vi "Draw Palette.vi"(2 "Bounds  Of Picture":T1, 3 "Display Data":T3[](array[typedef])) -> (0 "Co-ordinates":T2(array[cluster]), 1 "picture":picture)   [LabVIEW 2014, in "SmartPalette.lvlib"]
uses:
  SmartPalette.lvlib
  Controls/Palette Data.ctl
  <vilib>/picture/picture.llb/imagedata.ctl
  <vilib>/Utility/miscctls.llb/LVBoundsTypeDef.ctl
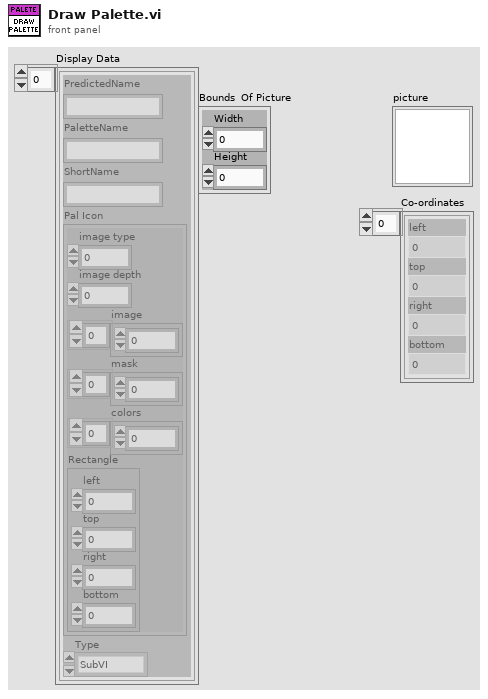
[diagram p1: front panel]
types:
  T1 = typedef "LVBoundsTypeDef.ctl" = cluster{"Width":u32, "Height":u32}
  T2 = cluster{"left":i16, "top":i16, "right":i16, "bottom":i16}[]
  T3 = typedef "SmartPalette.lvlib/Palette Data.ctl" = cluster{"PredictedName":string, "PaletteName":string, "ShortName":string, "Pal Icon":T4, "Type":enum16{"SubVI", "VI Templtate", "Function"}}
  T4 = typedef "imagedata.ctl" = cluster{"image type":i32, "image depth":i32, "image":u8[], "mask":u8[], "colors":u32[], "Rectangle":cluster{"left":i16, "top":i16, "right":i16, "bottom":i16}}
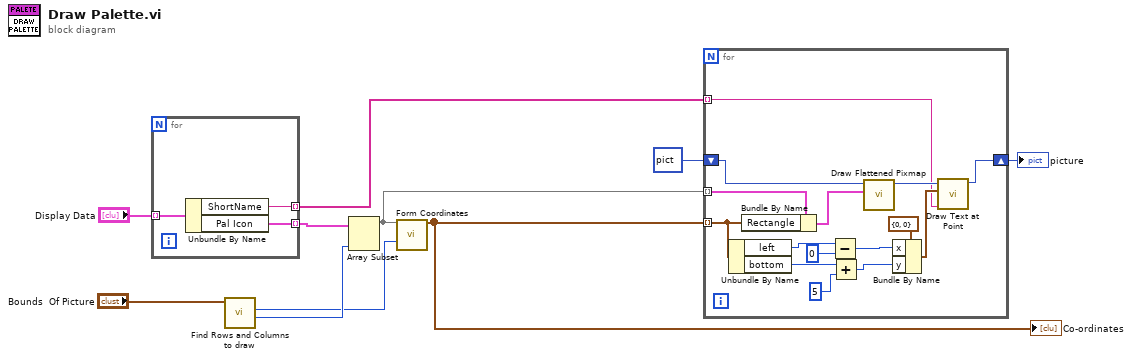
[diagram p0: block diagram]
diagram:
  n1 = for {
    tunnel: "Display Data" -> [w13] mode=indexing
    tunnel: [w12] -> w4 mode=indexing
    tunnel: [w11] -> w8 mode=indexing
    n2 = Unbundle By Name(w13) -> ("ShortName"=w11:string, "Pal Icon"=w12:T4)
  }
  n3 = call "Find Rows and Columns to draw.vi"("Bounds  Of Picture"="Bounds  Of Picture") -> ("Total"=w2:u32, "Col"=w1:u32)  [unwired: 8 in, 1 out]
  n4 = Array Subset(array=w4, length=w2) -> (w5:T4[])  [unwired: 1 in]
  n5 = call "Form Coordinates.vi"("Palette Item Icon"=w5, "No.of Elements in Row"=w1) -> ("Co-ordinates"=w6:T2)  [unwired: 13 in]
  "Co-ordinates" <- w6
  n6 = for {
    tunnel: w5 -> [w28] mode=indexing
    tunnel: w6 -> [w24] mode=indexing
    shift-right: [w20] -> w7
    shift-left: picture data[5B] ("picture") -> [w26]
    tunnel: w8 -> [w19] mode=indexing
    n7 = Unbundle By Name(w24) -> ("left"=w22:i16, "bottom"=w18:i16)
    n8 = Bundle By Name(cluster=w28, "Rectangle"=w24) -> (w27:T4)
    n9 = Subtract(x=w22, y=i16 0 ("x")) -> (x-y=w15:i16)
    n10 = Add(x=w18, y=i16 5) -> (x+y=w17:i16)
    n11 = call <vilib>:"Draw Flattened Pixmap.vi"("image data"=w27, "picture"=w26) -> ("new picture"=w25:picture)  [unwired: 7 in]
    n12 = Bundle By Name(cluster=cluster{"x":i16, "y":i16} {"x"=0, "y"=0} ("origin"), "x"=w15, "y"=w17) -> (w21:cluster{"x":i16, "y":i16})
    n13 = call <vilib>:"Draw Text at Point.vi"("text"=w19, "origin"=w21, "picture"=w25) -> ("new picture"=w20:picture)  [unwired: 7 in, 1 out]
  }
  "picture" <- w7
